vi "Tracer.vi"(8 "error in":errorcluster, 9 "Value":dbl, 10 "Operation Mode":enum16{"CC", "CV", "CP"}(ring), 11 "IT8800 Setting In In":T1={"VISA Resource Name"="", "Baud Rate"=19200, "Stop Bits"=20, "Wait For Read(ms)"=0} {"Stop Bits" items=["1.0"=10, "2.0"=20]; "Baud Rate" items=["2400"=2400, "4800"=4800, "9600"=9600, "19200"=19200]}) -> (0 "error out":errorcluster, 3 "IT8800 Setting In Out":T1={"VISA Resource Name"="", "Baud Rate"=19200, "Stop Bits"=20, "Wait For Read(ms)"=0} {"Stop Bits" items=["1.0"=10, "2.0"=20]; "Baud Rate" items=["2400"=2400, "4800"=4800, "9600"=9600, "19200"=19200]})   [LabVIEW 2018]
uses:
  Data Def/IT8800-Setting.ctl
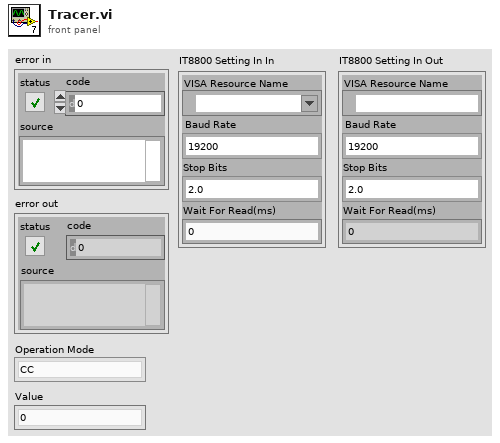
[diagram p1: front panel]
types:
  T1 = typedef "IT8800-Setting.ctl" = cluster{"VISA Resource Name":refnum<visa-resource-name>, "Baud Rate":u32, "Stop Bits":u16, "Wait For Read(ms)":u32}
  T2 = typedef "IT8800-Measurement Data.ctl" = cluster{"Current (Amps)":dbl, "Power (Watts)":dbl, "Voltage (Volts)":dbl, "Elapsed Time (Sec) ":dbl}
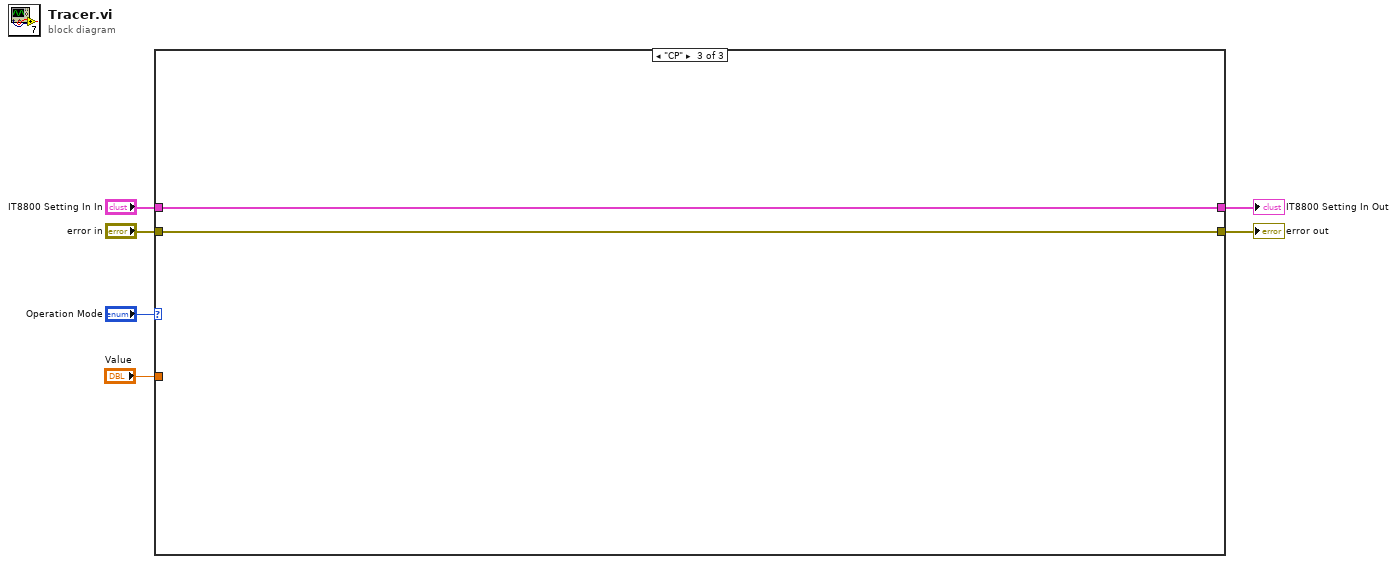
[diagram p0: block diagram]
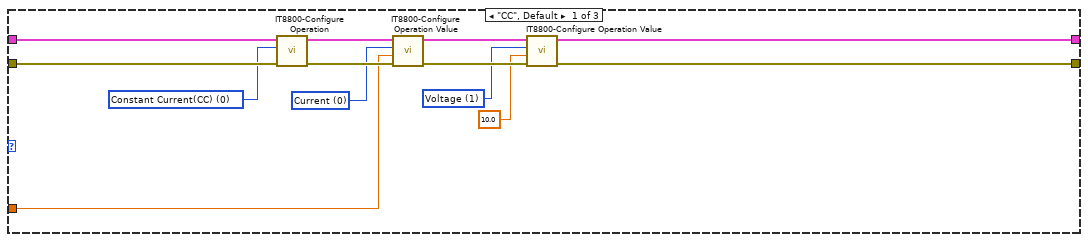
[diagram p2: hidden frame]
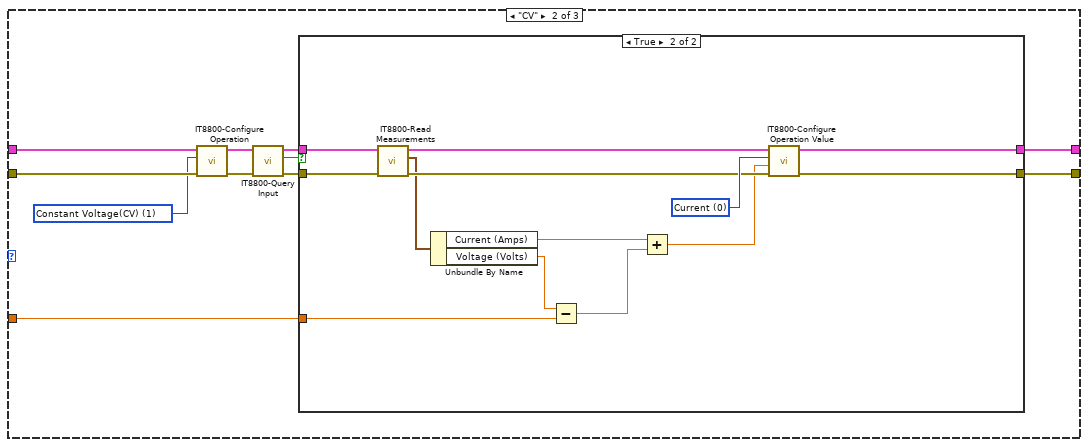
[diagram p3: hidden frame]
diagram:
  n1 = case shown="\"CP\"" "Operation Mode" {
    tunnel: "IT8800 Setting In In" -> [w19 w30 w46]
    tunnel: "error in" -> [w18 w29 w47]
    tunnel: "Value" -> [w13 w27 _]
    tunnel: [w9 w26 w46] -> w2
    tunnel: [w10 w25 w47] -> w1
    frame "CC", Default {
      w8 = u16 1 items=["Current", "Voltage", "Power", "Conductance"] ("Value Type (0:Current)")
      w14 = u16 0 items=["Current", "Voltage", "Power", "Conductance"] ("Value Type (0:Current)")
      w17 = u16 0 items=["Constant Current(CC)", "Constant Voltage(CV)", "Constant Power(CP)", "Constant Resistance(CR)", "Constant Current & Voltage(CCCV)", "Constant Resistance & Voltage(CRCV)"] ("Operation Mode (0:Constant Current)")
      n2 = call "IT8800-Configure Operation.vi"("error in"=w18, "Operation Mode (0:Constant Current)"=w17, "IT8800 Setting In In"=w19) -> ("error out"=w15:errorcluster, "IT8800 Setting In Out"=w16:T1)  [unwired: 7 in]
      n3 = call "IT8800-Configure Operation Value.vi"("error in"=w15, "Values (0)"=w13, "Value Type (0:Current)"=w14, "IT8800 Setting In In"=w16) -> ("error out"=w11:errorcluster, "IT8800 Setting In Out"=w12:T1)  [unwired: 6 in]
      n4 = call "IT8800-Configure Operation Value.vi"("error in"=w11, "Values (0)"=10.0, "Value Type (0:Current)"=w8, "IT8800 Setting In In"=w12) -> ("error out"=w10:errorcluster, "IT8800 Setting In Out"=w9:T1)  [unwired: 6 in]
    }
    frame "CV" {
      w28 = u16 1 items=["Constant Current(CC)", "Constant Voltage(CV)", "Constant Power(CP)", "Constant Resistance(CR)", "Constant Current & Voltage(CCCV)", "Constant Resistance & Voltage(CRCV)"] ("Operation Mode (0:Constant Current)")
      n5 = call "IT8800-Configure Operation.vi"("error in"=w29, "Operation Mode (0:Constant Current)"=w28, "IT8800 Setting In In"=w30) -> ("error out"=w24:errorcluster, "IT8800 Setting In Out"=w23:T1)  [unwired: 7 in]
      n6 = call "IT8800-Query Input.vi"("error in"=w24, "IT8800 Setting In In"=w23) -> ("error out"=w22:errorcluster, "Input?"=w20:bool, "IT8800 Setting In Out"=w21:T1)  [unwired: 7 in]
      n7 = case shown="True" w20 {
        tunnel: w27 -> [_ w36]
        tunnel: [w32 w44] -> w26
        tunnel: [w31 w43] -> w25
        tunnel: w22 -> [w31 w41]
        tunnel: w21 -> [w32 w42]
        frame False {
        }
        frame True {
          w45 = u16 0 items=["Current", "Voltage", "Power", "Conductance"] ("Value Type (0:Current)")
          n8 = call "IT8800-Read Measurements.vi"("error in"=w41, "IT8800 Setting In In"=w42) -> ("error out"=w39:errorcluster, "Measurement Data"=w38:T2, "IT8800 Setting In Out"=w40:T1)  [unwired: 7 in]
          n9 = Unbundle By Name(w38) -> ("Current (Amps)"=w35:dbl, "Voltage (Volts)"=w37:dbl)
          n10 = Subtract(x=w37, y=w36) -> (x-y=w33:dbl)
          n11 = Add(x=w35, y=w33) -> (x+y=w34:dbl)
          n12 = call "IT8800-Configure Operation Value.vi"("error in"=w39, "Values (0)"=w34, "Value Type (0:Current)"=w45, "IT8800 Setting In In"=w40) -> ("error out"=w43:errorcluster, "IT8800 Setting In Out"=w44:T1)  [unwired: 6 in]
        }
      }
    }
    frame "CP" {
    }
  }
  "error out" <- w1
  "IT8800 Setting In Out" <- w2
